vi "Untitled 2.vi"() -> ()   [LabVIEW 2018]
panel:
  out "curren":dbl
  in  "Step A":dbl
  in  "Min":dbl
  in  "Max":dbl
  out "REAL TIME":dbl
  in  "Tine":dbl
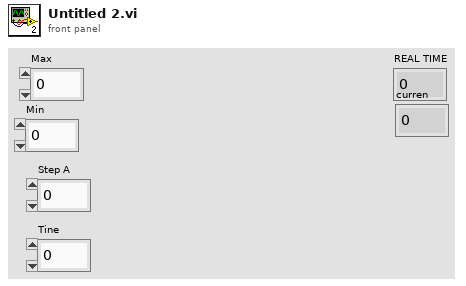
[diagram p1: front panel]
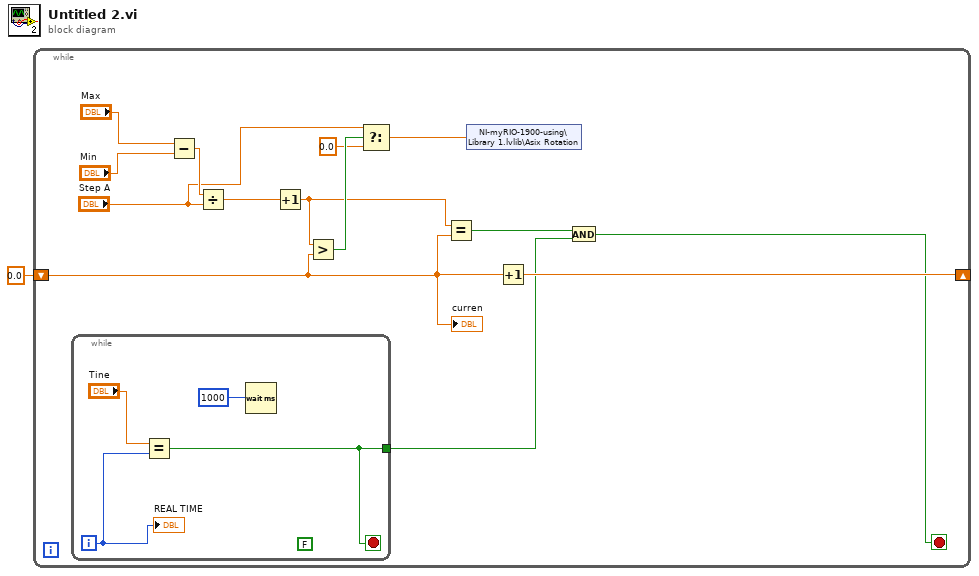
[diagram p0: block diagram]
diagram:
  n1 = while {
    shift-right: [w12] -> _
    shift-left: 0.0 -> [w5]
    stop <- w9 stop-if-true
    n2 = while {
      tunnel: [w16] -> w10
      i -> [w18]
      stop <- w16 stop-if-true
      (unwired) FALSE
      n3 = Equal?(x="Tine", y=w18) -> (x = y?=w16:bool)
      n4 = Wait (ms)(milliseconds to wait=u32 1000) -> ()  [unwired: 1 out]
      "REAL TIME" <- w18
    }
    n5 = Subtract(x="Max", y="Min") -> (x-y=w13:dbl)
    n6 = Divide(x=w13, y="Step A") -> (x/y=w8:dbl)
    n7 = Increment(x=w8) -> (x+1=w6:dbl)
    n8 = Greater?(x=w6, y=w5) -> (0:w7:bool)
    n9 = Select(t="Step A", s=w7, f=0.0) -> (s? t:f=w2:dbl)
    n10 = Equal?(x=w6, y=w5) -> (x = y?=w11:bool)
    n11 = shared-variable "NI-myRIO-1900-using\\Library 1.lvlib\\Asix Rotation"(w2) -> ()  [unwired: 1 in, 1 out]
    n12 = Increment(x=w5) -> (x+1=w12:dbl)
    n13 = And(x=w11, y=w10) -> (x .and. y?=w9:bool)
    "curren" <- w5
  }
